vi "Hybrid Connect.vi"(0 "VI Name":string) -> (1 "VI Refnum":refnum<vi>, 2 "Success":bool, 3 "error out":errorcluster)   [LabVIEW 2020]
uses:
  Sub Controls/LV Versions Enum.ctl
panel:
  out "Target LV Version #":T1
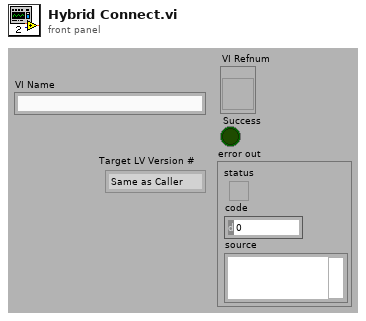
[diagram p1: front panel]
types:
  T1 = typedef "LV Versions Enum.ctl" = enum16{"Same as Caller", "8.0", "8.20", "8.5", "8.6", "9.0", "10.0", "11.0", "12.0", "13.0", "14.0", "15.0", "16.0", "17.0", "18.0", "19.0", "20.0"}
  T2 = enum32{"Bad", "Idle", "Run top level", "Running"}
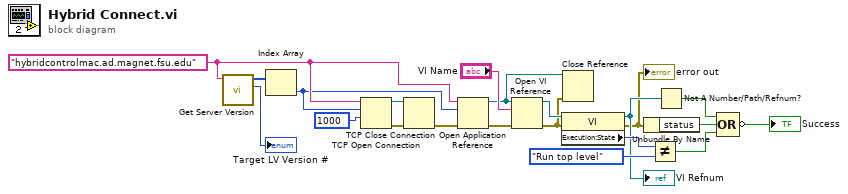
[diagram p0: block diagram]
diagram:
  w5 = "hybridcontrolmac.ad.magnet.fsu.edu" ("machine name (\"\":  open local reference)")
  n1 = call "Get Server Version.vi"("Machine Name"=w5) -> ("Target LV Version #"=→"Target LV Version #":T1, "Open LabVIEW Ports"=w3:u16[])  [unwired: 8 in, 1 out]
  n2 = Index Array(array=w3) -> (element=w2:u16)  [unwired: 1 in]
  n3 = TCP Open Connection(address=w5, remote port or service name=w2, timeout ms (60000)=1000) -> (connection ID=w19:refnum<k5>, error out=w20:errorcluster)  [unwired: 2 in]
  n4 = TCP Close Connection(connection ID=w19, error in (no error)=w20) -> (error out=w21:errorcluster)  [unwired: 1 in, 1 out]
  n5 = Open Application Reference(8:w21, 10:w2, 11:w5) -> (0:w18:errorcluster, 3:w13:refnum<vi>)  [unwired: 1 in]
  n6 = Open VI Reference(application reference (local)=w13, vi path="VI Name", error in (no error)=w18) -> (vi reference=w10:refnum<vi>, error out=w7:errorcluster)  [unwired: 3 in]
  n7 = property class="VI"(reference=w10, error in=w7) -> (reference out=w9:refnum<vi>, error out=w8:errorcluster, "Execution:State"=w11:T2)
  "error out" <- w8
  "VI Refnum" <- w9
  n8 = Close Reference(reference=w13, error in (no error)=w7) -> ()  [unwired: 1 out]
  n9 = Unbundle By Name(w8) -> ("status"=w15:bool)
  n10 = Not Equal?(x=w11, y=T2."Run top level" ("Execution:State")) -> (x != y?=w6:bool)
  n11 = Not A Number/Path/Refnum?(number/path/refnum=w9) -> (NaN/Path/Refnum?=w16:bool)
  n12 = Compound Arithmetic op=OR(w16, w15, w6) -> (invert →"Success":bool)
